vi "PH_ImageCalibrator.constructor.vi"(0 "name":string, 2 "data in":string, 5 "error in":errorcluster) -> (14 "i ref out":refnum<vi>, 16 "data out":string, 19 "error out":errorcluster)   [LabVIEW 2014, in "PH_ImageCalibrator.lvlib"]
doc: "This class takes and stores several beam profile settings. This is relevant for the class PH_ImageOperator.\n\nThis class is part of the PHELIX user layer.\n\nauthor: Stefan Götte, GSI\n\nLicense Agreement for this software:\n\nCopyright (C)\nGesellschaft für Schwerionenforschung, GSI\nPlanckstr. 1\n64291 Darmstadt\nGermany\n\nContact: D.Beck@gsi.de \n\nThis program is free software; you can redistribute it and/or modify it under the terms of the \nGNU General Public License as published by the Free Software Foundation; either version 2 of \nthe license, or (at your option) any later version.\n\nThis program is distributed in the hope that it will be useful, but WITHOUT ANY WARRANTY; \nwithout even the implied warranty of MERCHANTABILITY or FITNESS FOR A PARTICULAR PURPOSE. See the GNU General License for more details (http://www.gnu.org).\n\nGesellschaft für Schwerionenforschung, GSI\nPlanckstr. 1, 64291 Darmstadt, Germany\nFor all questions and ideas contact: M.Richter@gsi.de, H.Brand@gsi.de or D.Beck@gsi.de.\nLast update: 16-JUN-2004"
uses:
  PH_ImageCalibrator.lvlib
  PH_Img_BaseClass/PH_Img_BaseClass.Palette.ctl
  CSCore/CSObj/CSObj.lvlib
  PH_Img_BaseClass/PH_Img_BaseClass.lvlib
  PH_Common/PH_Common.lvlib
  PH_Class/PH_Class.lvlib
  PH_SM_Class/PH_SM_Class.lvlib
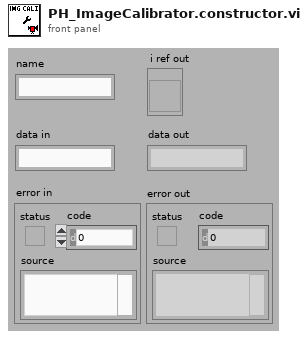
[diagram p1: front panel]
types:
  T1 = enum16{"SetAttribute", "GetAttribute", "CreateAttribute", "DestroyAttribute", "DestroyAllAtributes"}
  T2 = typedef "PH_Img_BaseClass.lvlib/PH_Img_BaseClass.Palette.ctl" = i32
  T3 = typedef "PH_ImageCalibrator.lvlib/PH_ImageCalibrator.i attribute.ctl" = cluster{"GUI Refs":cluster{"Available Cams":refnum<vi>, "OK":refnum<vi>, "Skip":refnum<vi>, "Repeat":refnum<vi>, "Cancel":refnum<vi>, "Length [mm]":refnum<vi>, "Energy [mJ]":refnum<vi>, "Dialog":refnum<vi>}, "Cam instances":string[], "Dark Pics":cluster{"#":i32, "BI taken":bool}, "Lin Cali":cluster{"Distance [Pixel]":dbl, "Distance [mm]":dbl, "Lin Cali Factor [mm/Pixel]":dbl}, "Energy Cali":cluster{"Pixelsum":dbl, "Energy [mJ]":dbl, "Energy Cali factor [mJ/Pixelsum]":dbl, "Underground subtracted?":bool, "#":i32}, "Images":cluster{"Background":T4, "Energy":T4}}
  T4 = typedef "IMAQ Image.ctl" = refnum<image>
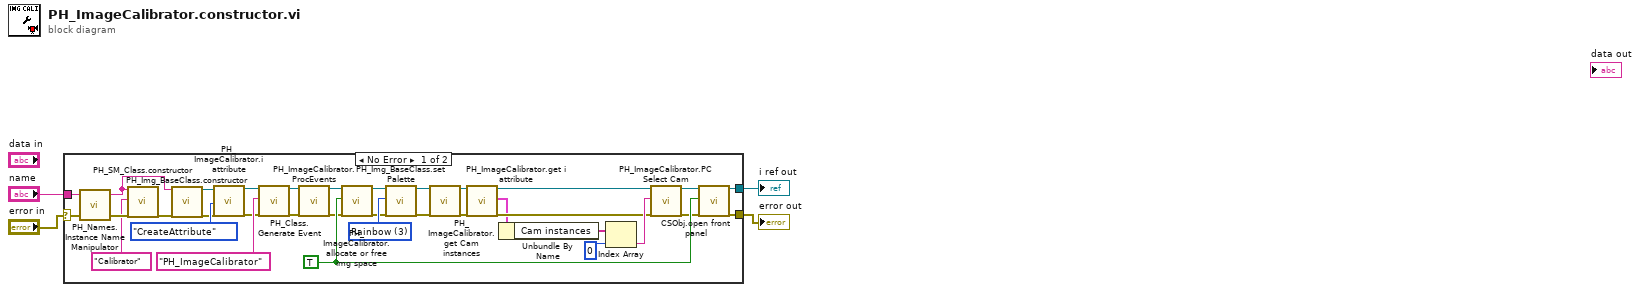
[diagram p0: block diagram]
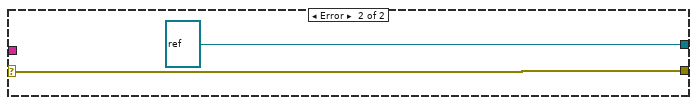
[diagram p2: hidden frame]
diagram:
  n1 = case shown="No Error" "error in" {
    selector: "error in" -> [w35 w39]
    tunnel: "name" -> [w34 _]
    tunnel: [w8 refnum<vi> refnum ("i ref out")] -> w3
    tunnel: [w7 w39] -> w2
    frame No Error {
      w36 = T2 3 items=["Grey", "Binary", "Gradient", "Rainbow", "Temperature"] ("Palette")
      w38 = TRUE ("front panel open")
      n2 = call "PH_Names.Instance Name Manipulator.vi"("error in (no error)"=w35, "name in"=w34) -> ("error out"=w28:errorcluster, "name out"=w25:string)  [unwired: 1 in, 1 out]
      n3 = call "PH_SM_Class.constructor.vi"("name"=w25, "data in"="Calibrator" ("object"), "error in"=w28) -> ("error out"=w27:errorcluster)  [unwired: 14 in, 2 out]
      n4 = call "PH_Img_BaseClass.constructor.vi"("name"=w25, "error in(no error)"=w27) -> ("i ref out"=w32:refnum<vi>, "error out"=w33:errorcluster)  [unwired: 15 in, 1 out]
      n5 = call "PH_ImageCalibrator.i attribute.vi"("VI Refnum"=w32, "Action"=T1."CreateAttribute", "error in (no error)"=w33) -> ("VI Refnum out"=w30:refnum<vi>, "error out"=w29:errorcluster)  [unwired: 14 in, 1 out]
      n6 = call "PH_Class.Generate Event.vi"("i ref in"=w30, "Class"="PH_ImageCalibrator", "error in (no error)"=w29) -> ("i ref out"=w23:refnum<vi>, "error out"=w24:errorcluster)  [unwired: 15 in]
      n7 = call "PH_ImageCalibrator.ProcEvents.vi"("i ref in"=w23, "error in"=w24) -> ("i ref out"=w22:refnum<vi>, "error out"=w21:errorcluster)  [unwired: 16 in]
      n8 = call "PH_ImageCalibrator.allocate or free img space.vi"("i ref in"=w22, "Allocate?"=w38, "error in (no error)"=w21) -> ("i ref out"=w20:refnum<vi>, "error out"=w19:errorcluster)  [unwired: 15 in]
      n9 = call "PH_Img_BaseClass.set Palette.vi"("i ref in"=w20, "Palette"=w36, "error in (no error)"=w19) -> ("i ref out"=w6:refnum<vi>, "error out"=w5:errorcluster)  [unwired: 15 in]
      n10 = call "PH_ImageCalibrator.get Cam instances.vi"("i ref in"=w6, "error in"=w5) -> ("i ref out"=w11:refnum<vi>, "error out"=w12:errorcluster)  [unwired: 16 in]
      n11 = call "PH_ImageCalibrator.get i attribute.vi"("i ref in"=w11, "error in (no error)"=w12) -> ("i ref out"=w16:refnum<vi>, "i attribute"=w13:T3, "error out"=w17:errorcluster)  [unwired: 15 in]
      n12 = Unbundle By Name(w13) -> ("Cam instances"=w14:string[])
      n13 = Index Array(array=w14, index=0) -> (element=w18:string)
      n14 = call "PH_ImageCalibrator.PC Select Cam.vi"("VI in"=w16, "Source"=w18, "error in (no error)"=w17) -> ("VI out"=w10:refnum<vi>, "error out"=w9:errorcluster)  [unwired: 15 in]
      n15 = call "CSObj.open front panel.vi"("i ref in"=w10, "frontPanelOpen"=w38, "error in (no error)"=w9) -> ("i ref out"=w8:refnum<vi>, "error out"=w7:errorcluster)  [unwired: 15 in]
    }
    frame Error {
    }
  }
  "i ref out" <- w3
  "error out" <- w2
